vi "Start_Stop Polling Mode.vi"(8 "error in":errorcluster, 10 "Star Polling?":bool, 11 "Neph in":refnum<class "Nephelometer.lvclass">) -> (0 "error out":errorcluster, 3 "Neph out":refnum<class "Nephelometer.lvclass">)   [LabVIEW 2014, in "Nephelometer.lvclass"]
uses:
  Nephelometer.lvclass
  Reusable/Session APIs/Serial/Serial Session.lvclass
  Nephelometer.lvclass/Nephelometer.ctl
  Accessors/Read Session Handle.vi
  <userlib>/_Session Fwk/Session - Root.lvclass
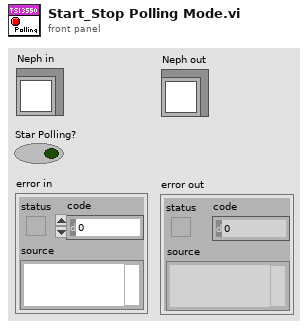
[diagram p1: front panel]
types:
  T1 = typedef "Session - Root.lvclass/Session Handle.ctl" = refnum<data-value>
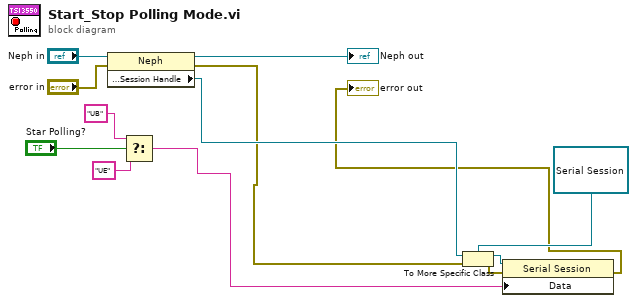
[diagram p0: block diagram]
diagram:
  n1 = property class="Neph"(reference="Neph in", error in="error in") -> (reference out=→"Neph out":refnum<class "Nephelometer.lvclass">, error out=w3:errorcluster, "Accessors:Session Handle"=w6:T1)
  n2 = Select(t="UB" ("Write - Asynchronous"), s="Star Polling?", f="UE" ("Write - Asynchronous")) -> (s? t:f=w4:string)
  n3 = To More Specific Class(target class=refnum<data-value> refnum ("Session Handle"), reference=w6, error in=w3) -> (specific class reference=w5:refnum<data-value>, error out=w2:errorcluster)
  n4 = property class="Serial Session"(reference=w5, error in=w2, "Data"=w4) -> (error out=→"error out":errorcluster)  [unwired: 1 out]
